vi "niRFUtil RFHS Math Apply Polynomial SGL.vi"(0 "X":sgl[](array[numeric]), 5 "P(A)":sgl[](array[numeric]) min=0 max=127 format="%.2f", 11 "error in":errorcluster) -> (4 "P(x)":sgl[](array[numeric]) min=0 max=127 format="%.2f", 15 "error out":errorcluster)   [LabVIEW 2015, in "niRFUtil.lvlib"]
uses:
  niRFUtil.lvlib
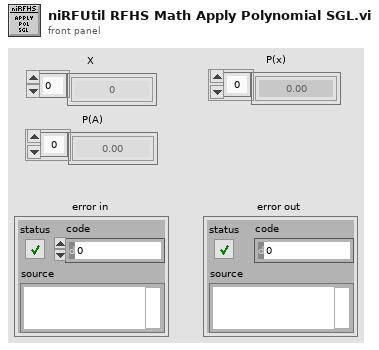
[diagram p1: front panel]
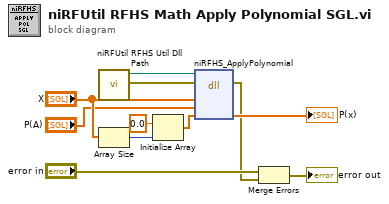
[diagram p0: block diagram]
diagram:
  n1 = call "niRFUtil RFHS Util Dll Path.vi"() -> ("error out"=w2:errorcluster, "Path"=w4:path)  [unwired: 7 in, 3 out]
  n2 = Array Size(array="X") -> (size(s)=w5:i32)
  n3 = Initialize Array(sgl 0.0 ("Numeric"), w5) -> (w3:sgl[])
  n4 = dll-call lib="R:/niRFHS.dll" fn="niRFHS_ApplyPolynomial"(path in=w4, error in=w2, "input"="X", "polynom"="P(A)", "output"=w3) -> (error out=w1:errorcluster, "output"=→"P(x)":sgl[])  [unwired: 4 in, 1 out]
  n5 = Merge Errors("error in", w1) -> (→"error out":errorcluster)
